vi "Report - Parse Data to TDMS (SubVI).vi"(8 "error in (no error)":errorcluster, 11 "Cluster":T1) -> (0 "error out":errorcluster, 3 "Cancel?":bool)   [LabVIEW 2019]
uses:
  Controls/Report - Data Structure.ctl
  <vilib>/httpClient/ClientHandle.ctl
  Controls/JSON - GetData.ctl
  <vilib>/httpClient/POSTBuffer.vi
  <vilib>/httpClient/LabVIEWHTTPClient.lvlib
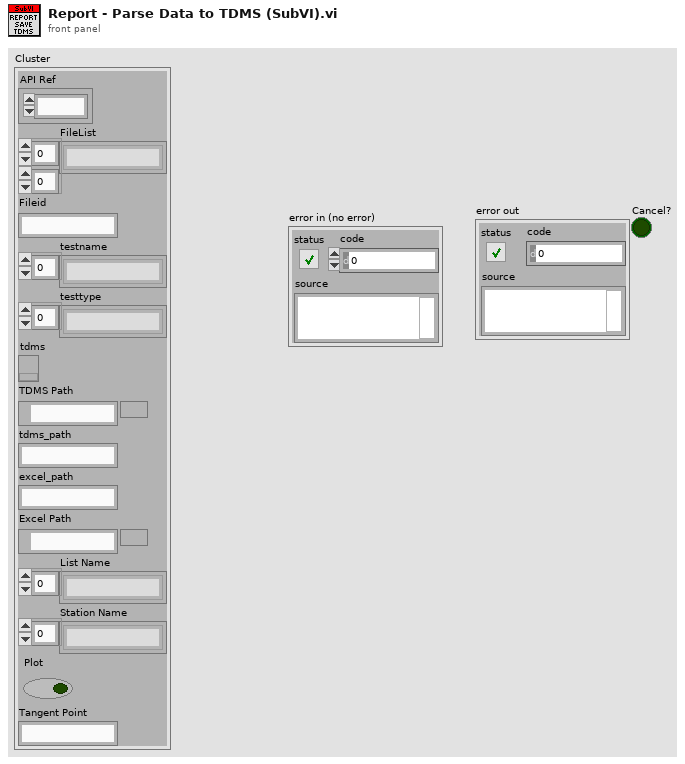
[diagram p1: front panel]
types:
  T1 = typedef "Report - Data Structure.ctl" = cluster{"API Ref":T2, "FileList":string[][], "Fileid":string, "testname":string[], "testtype":string[], "tdms":refnum<k34>, "TDMS Path":path, "tdms_path":string, "excel_path":string, "Excel Path":path, "List Name":string[], "Station Name":string[], "Plot":bool, "Tangent Point":string}
  T2 = typedef "LabVIEWHTTPClient.lvlib/ClientHandle.ctl" = refnum<k1>
  T3 = cluster{"status":string, "data":cluster{"id":string, "created_date":string, "testname":string, "jobno":string, "jobdesc":string, "sampleid":string, "date":string, "specimentno":string, "depth":string, "height":string, "diameter":string, "weight":string, "done":string}[]}
  T4 = cluster{"id":string, "created_date":string, "testname":string, "jobno":string, "jobdesc":string, "sampleid":string, "date":string, "specimentno":string, "depth":string, "height":string, "diameter":string, "weight":string, "done":string}[]
  T5 = cluster{"id":string, "created_date":string, "testname":string, "jobno":string, "jobdesc":string, "sampleid":string, "date":string, "specimentno":string, "depth":string, "height":string, "diameter":string, "weight":string, "done":string}
  T6 = cluster{"testtype":u16, "testname":string, "fileid":string}
  T7 = typedef "JSON - GetData.ctl" = cluster{"status":string, "data":cluster{"timestamp":string, "elapsetime":string, "testname":string, "testtype":u16, "data":string[]}[]}
  T8 = cluster{"timestamp":string, "elapsetime":string, "testname":string, "testtype":u16, "data":string[]}[]
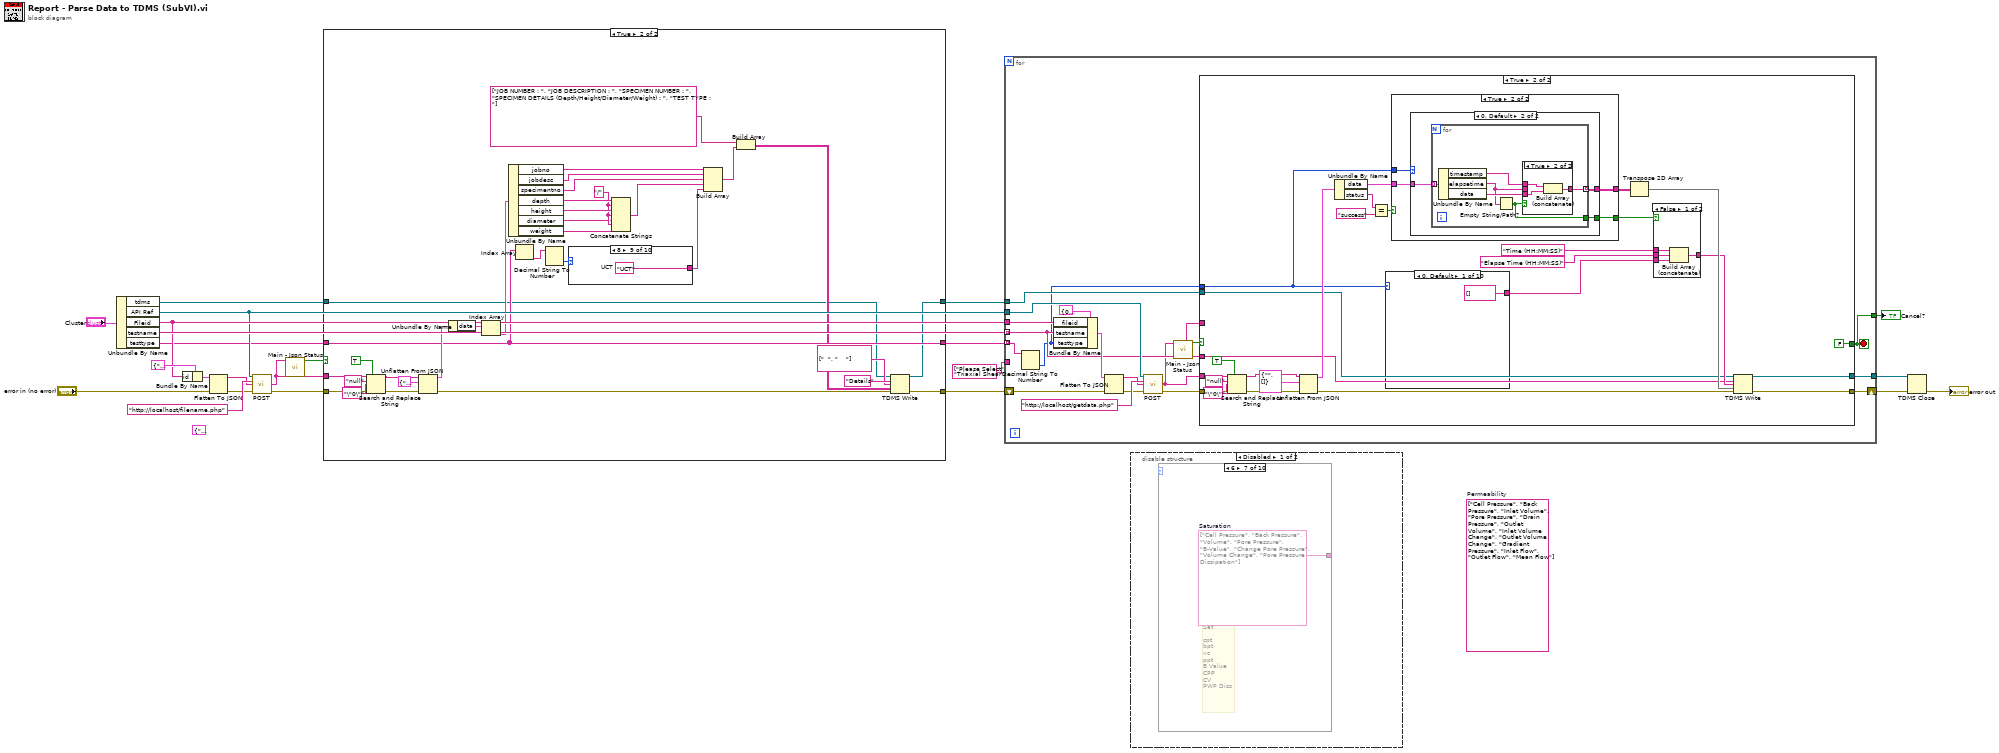
[diagram p0: block diagram]
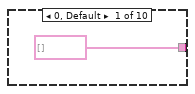
[diagram p2: hidden frame]
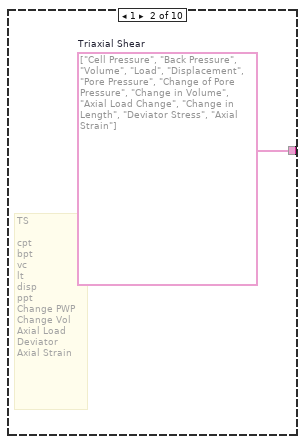
[diagram p3: hidden frame]
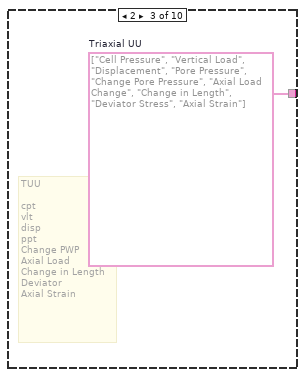
[diagram p4: hidden frame]
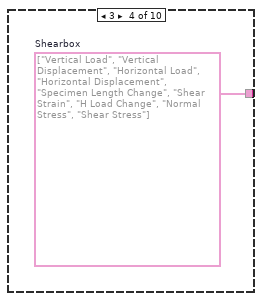
[diagram p5: hidden frame]
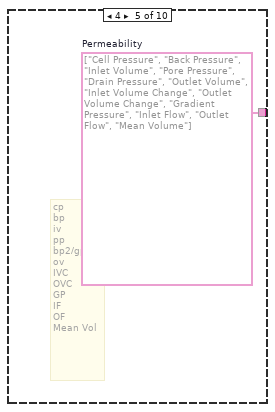
[diagram p6: hidden frame]
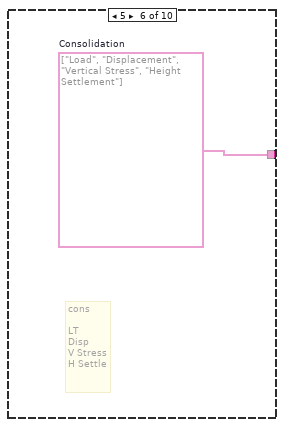
[diagram p7: hidden frame]
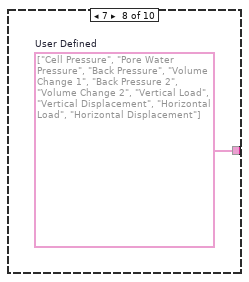
[diagram p8: hidden frame]
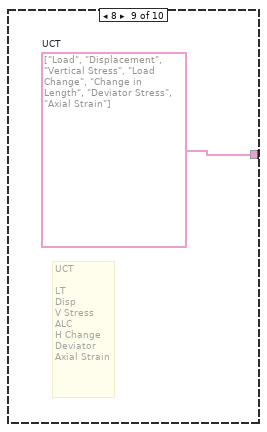
[diagram p9: hidden frame]
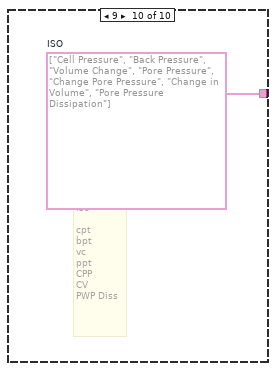
[diagram p10: hidden frame]
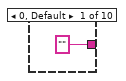
[diagram p13: hidden frame]
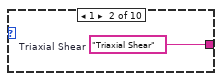
[diagram p14: hidden frame]
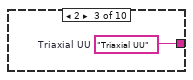
[diagram p15: hidden frame]
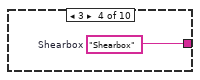
[diagram p16: hidden frame]
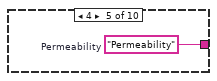
[diagram p17: hidden frame]
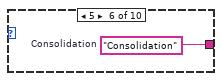
[diagram p18: hidden frame]
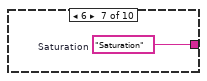
[diagram p19: hidden frame]
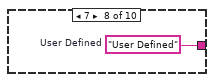
[diagram p20: hidden frame]
diagram:
  (unwired) string[] ["Cell Pressure", "Back Pressure", "Inlet Volume", "Pore Pressure", "Drain Pressure", "Outlet Volume", "Inlet Volume Change", "Outlet Volume Change", "Gradient Pressure", "Inlet Flow", "Outlet Flow", "Mean Flow"]  # Permeability
  (unwired) cluster{"action":string} {"action"="read_all"}
  n1 = Unbundle By Name("Cluster") -> ("tdms"=w4:refnum<k34>, "API Ref"=w5:T2, "Fileid"=w10:string, "testname"=w21:string[], "testtype"=w3:string[])
  n2 = Bundle By Name(cluster=cluster{"action":string, "id":string} {"action"="read_by_id", "id"="2"}, "id"=w10) -> (w14:cluster{"action":string, "id":string})
  n3 = Flatten To JSON(anything=w14, error in (no error)="error in (no error)") -> (JSON string=w15:string, 11:w12:errorcluster)  [unwired: 1 in]
  n4 = call-poly <vilib>:"POST.vi"("client handle"=w5, "url"="http://localhost/filename.php", "buffer"=w15, "error in (no error)"=w12) -> ("body"=w7:string, "error out"=w8:errorcluster)  [unwired: 8 in, 2 out]
  n5 = call "Main - Json Status.vi"("json"=w7) -> ("Success?"=w6:bool)  [unwired: 9 in, 1 out]
  n6 = case shown="True" w6 {
    tunnel: [w26 w32] -> w9
    tunnel: w8 -> [w26 w55]
    tunnel: w7 -> [_ w53]
    tunnel: w4 -> [w24 w27]
    tunnel: w3 -> [w25 w48]
    tunnel: [w24 w31] -> w2
    tunnel: [w25 w48] -> w1
    frame False {
    }
    frame True {
      w45 = "/" ("string")
      n7 = Search and Replace String(replace all?=TRUE ("replace all? (F)"), input string=w53, search string="null", replace string="\"0\"" ("replace string (\"\")"), error in=w55) -> (result string=w52:string, error out=w54:errorcluster)  [unwired: 3 in, 2 out]
      n8 = Unflatten From JSON(JSON string=w52, type and defaults=T3 {"status"="read_all", "data"=[]}, error in (no error)=w54) -> (value=w51:T3, error out=w33:errorcluster)  [unwired: 4 in]
      n9 = Unbundle By Name(w51) -> ("data"=w50:T4)
      n10 = Index Array(array=w50) -> (element=w49:T5)  [unwired: 1 in]
      n11 = Unbundle By Name(w49) -> ("jobno"=w40:string, "jobdesc"=w39:string, "specimentno"=w38:string, "depth"=w47:string, "height"=w46:string, "diameter"=w44:string, "weight"=w43:string)
      n12 = Index Array(array=w48) -> (element=w42:string)  [unwired: 1 in]
      n13 = Decimal String To Number(string=w42) -> (number=w41:i32)  [unwired: 2 in, 1 out]
      n14 = case shown="8" w41 {
        tunnel: ["" w61 w62 w63 w64 w65 w66 w67 w68 w69] -> w36
        frame 0, Default {
        }
        frame 1 {
          w61 = "Triaxial Shear"  # Triaxial Shear
        }
        frame 2 {
          w62 = "Triaxial UU"  # Triaxial UU
        }
        frame 3 {
          w63 = "Shearbox"  # Shearbox
        }
        frame 4 {
          w64 = "Permeability"  # Permeability
        }
        frame 5 {
          w65 = "Consolidation"  # Consolidation
        }
        frame 6 {
          w66 = "Saturation"  # Saturation
        }
        frame 7 {
          w67 = "User Defined"  # User Defined
        }
        frame 8 {
          w68 = "UCT"  # UCT
        }
        frame 9 {
          w69 = "Iso Consolidation"  # Iso
        }
      }
      n15 = Concatenate Strings(w47, w45, w46, w45, w44, w45, w43) -> (w37:string)
      n16 = Build Array(w40, w39, w38, w37, w36) -> (w34:string[])
      n17 = Build Array(string[] ["JOB NUMBER : ", "JOB DESCRIPTION : ", "SPECIMEN NUMBER : ", "SPECIMEN DETAILS (Depth/Height/Diameter/Weight) : ", "TEST TYPE : "], w34) -> (w28:string[][])
      n18 = TDMS Write(0:w27, 5:"Details" ("group name in (Untitled)"), 7:string[] ["  ", "    "] ("channel name(s) in (Untitled)"), 9:w28, 11:w33) -> (4:w31:refnum<k34>, 15:w32:errorcluster)  [unwired: 1 in, 2 out]
    }
  }
  n19 = for {
    tunnel: w21 -> [w79] mode=indexing
    tunnel: w1 -> [w75] mode=indexing
    tunnel: w10 -> [w86]
    tunnel: w5 -> [w81]
    tunnel: string[] ["Please Select", "Triaxial Shear", "Triaxial UU", "Shearbox", "Permeability", "Consolidation", "Saturation", "User Defined"] ("Strings []") -> [_]
    shift-right: [w78] -> w20
    shift-left: w9 -> [w85]
    tunnel: w2 -> [w80]
    tunnel: [w77] -> w18
    tunnel: [w70] -> w17
    stop <- w70 stop-if-true
    n20 = Decimal String To Number(string=w75) -> (number=w74:i32)  [unwired: 2 in, 1 out]
    n21 = Bundle By Name(cluster=T6 {"testtype"=0, "testname"="", "fileid"=""}, "fileid"=w86, "testname"=w79, "testtype"=w74) -> (w87:T6)
    n22 = Flatten To JSON(anything=w87, error in (no error)=w85) -> (JSON string=w82:string, 11:w83:errorcluster)  [unwired: 1 in]
    n23 = call-poly <vilib>:"POST.vi"("client handle"=w81, "url"="http://localhost/getdata.php", "buffer"=w82, "error in (no error)"=w83) -> ("body"=w73:string, "error out"=w76:errorcluster)  [unwired: 8 in, 2 out]
    n24 = call "Main - Json Status.vi"("json"=w73) -> ("Success?"=w72:bool, "message"=w71:string)  [unwired: 9 in]
    n25 = case shown="True" w72 {
      tunnel: w80 -> [w96 w112]
      tunnel: w79 -> [_ w111]
      tunnel: [w97 w110] -> w78
      tunnel: [w96 w99] -> w77
      tunnel: w76 -> [w97 w109]
      tunnel: w74 -> [_ w98]
      tunnel: w73 -> [w92 w103]
      tunnel: w71 -> [w89 _]
      tunnel: [w93 FALSE ("T button?")] -> w70
      frame False {
        n26 = Concatenate Strings(w92, " " ("string"), w89) -> (w90:string)
        n27 = Two Button Dialog(message=w90, 1:"Proceed without this data" ("F button name (\"Cancel\")"), 2:"Cancel report generation" ("T button name (\"OK\")")) -> (T button?=w93:bool)
      }
      frame True {
        n28 = Search and Replace String(replace all?=TRUE ("replace all? (F)"), input string=w103, search string="null", replace string="\"0\"" ("replace string (\"\")"), error in=w109) -> (result string=w107:string, error out=w108:errorcluster)  [unwired: 3 in, 2 out]
        n29 = Unflatten From JSON(JSON string=w107, type and defaults=T7 {"status"="", "data"=[]}, error in (no error)=w108) -> (value=w119:T7, error out=w113:errorcluster)  [unwired: 4 in]
        n30 = Unbundle By Name(w119) -> ("data"=w122:T8, "status"=w121:string)
        n31 = Equal?(x=w121, y="success") -> (x = y?=w123:bool)
        n32 = case shown="0, Default" w98 {
          tunnel: [string[] [] w133 w134 w135 w136 w137 w138 w139 w140 w141] -> w100
          frame 0, Default {
          }
          frame 1 {
            w133 = string[] ["Cell Pressure", "Back Pressure", "Volume Change", "Load", "Displacement", "Pore Pressure", "Change of Pore Pressure", "Change in Volume", "Axial Load Change", "Change in Length", "Deviator Stress", "Axial Strain"]  # Triaxial Shear
          }
          frame 2 {
            w134 = string[] ["Cell Pressure", "Vertical Load", "Displacement", "Pore Pressure", "Change Pore Pressure", "Axial Load Change", "Change in Length", "Deviator Stress", "Axial Strain"]  # Triaxial UU
          }
          frame 3 {
            w135 = string[] ["Vertical Load", "Vertical Displacement", "Horizontal Load", "Horizontal Displacement", "Specimen Length Change", "Shear Strain", "H Load Change", "Normal Stress", "Shear Stress"]  # Shearbox
          }
          frame 4 {
            w136 = string[] ["Cell Pressure", "Back Pressure", "Inlet Volume", "Pore Pressure", "Drain Pressure", "Outlet Volume", "Inlet Volume Change", "Outlet Volume Change", "Gradient Pressure", "Inlet Flow", "Outlet Flow", "Mean Flow"]  # Permeability
          }
          frame 5 {
            w137 = string[] ["Load", "Displacement", "Vertical Stress", "Height Settlement", "Total Height Settlement"]  # Consolidation
          }
          frame 6 {
            w138 = string[] ["Cell Pressure", "Back Pressure", "Sample Volume", "Pore Pressure", "B-Value", "Pore Pressure Change", "Sample Volume Change"]  # Saturation
          }
          frame 7 {
            w139 = string[] ["Cell Pressure", "Pore Water Pressure", "Back Pressure", "Volume Change 1", "Back Pressure 2", "Volume Change 2", "Vertical Load", "Vertical Displacement", "Horizontal Load", "Horizontal Displacement"]  # User Defined
          }
          frame 8 {
            w140 = string[] ["Load", "Displacement", "Vertical Stress", "Load Change", "Change in Length", "Deviator Stress", "Axial Strain"]  # UCT
          }
          frame 9 {
            w141 = string[] ["Cell Pressure", "Back Pressure", "Sample Volume", "Pore Pressure", "Pore Pressure Change", "Sample Volume Change", "Pore Pressure Dissipation"]  # Iso
          }
        }
        n33 = case shown="True" w123 {
          tunnel: w122 -> [_ w147]
          tunnel: [string[][] [] w146] -> w115
          tunnel: [FALSE w145] -> w117
          tunnel: w98 -> [_ w144]
          frame False {
          }
          frame True {
            n34 = case shown="0, Default" w144 {
              tunnel: w147 -> [w151 w172]
              tunnel: [w150 w171] -> w146
              tunnel: [w149 w170] -> w145
              frame 5 {
                n35 = for {
                  tunnel: w151 -> [w160] mode=indexing
                  tunnel: [w158] -> w150 mode=indexing if=w153
                  tunnel: [w157] -> w149
                  shift-right: [w154] -> _
                  shift-left: "" -> [w155]
                  n36 = Unbundle By Name(w160) -> ("timestamp"=w159:string, "elapsetime"=w154:string, "data"=w156:string[])
                  n37 = Empty String/Path?(string/path=w154) -> (empty?=w157:bool)
                  n38 = Not Equal?(x=w155, y=w154) -> (x != y?=w152:bool)
                  n39 = case shown="False" w157 {
                    tunnel: w159 -> [w165 w169]
                    tunnel: w156 -> [w162 w167]
                    tunnel: [w164 w168] -> w158
                    tunnel: w154 -> [w163 _]
                    tunnel: [w161 TRUE] -> w153
                    tunnel: w152 -> [w161 _]
                    frame False {
                      n40 = Build Array (concatenate)(w165, w163, w162) -> (w164:string[])
                    }
                    frame True {
                      n41 = Build Array (concatenate)(w169, w167) -> (w168:string[])
                    }
                  }
                }
              }
              frame 0, Default {
                n42 = for {
                  tunnel: w172 -> [w178] mode=indexing
                  tunnel: [w176] -> w171 mode=indexing
                  tunnel: [w175] -> w170
                  n43 = Unbundle By Name(w178) -> ("timestamp"=w177:string, "elapsetime"=w173:string, "data"=w174:string[])
                  n44 = Empty String/Path?(string/path=w173) -> (empty?=w175:bool)
                  n45 = case shown="True" w175 {
                    tunnel: w177 -> [w182 w185]
                    tunnel: w174 -> [w179 w183]
                    tunnel: [w181 w184] -> w176
                    tunnel: w173 -> [w180 _]
                    frame False {
                      n46 = Build Array (concatenate)(w182, w180, w179) -> (w181:string[])
                    }
                    frame True {
                      n47 = Build Array (concatenate)(w185, w183) -> (w184:string[])
                    }
                  }
                }
              }
            }
          }
        }
        n48 = Transpose 2D Array(2D array=w115) -> (transposed array=w116:string[][])
        n49 = case shown="False" w117 {
          tunnel: "Time (HH:MM:SS)" ("element") -> [w128 w131]
          tunnel: w100 -> [w125 w129]
          tunnel: [w127 w130] -> w114
          tunnel: "Elapse Time (HH:MM:SS)" ("String") -> [w126 _]
          frame False {
            n50 = Build Array (concatenate)(w128, w126, w125) -> (w127:string[])
          }
          frame True {
            n51 = Build Array (concatenate)(w131, w129) -> (w130:string[])
          }
        }
        n52 = TDMS Write(0:w112, 5:w111, 7:w114, 9:w116, 11:w113) -> (4:w99:refnum<k34>, 15:w110:errorcluster)  [unwired: 1 in, 2 out]
      }
    }
  }
  "Cancel?" <- w17
  n53 = disable-structure shown="Disabled" {
    frame Disabled {
      n54 = case shown="6" {
        selector: _ -> [_ _ _ _ _ _ _ _ _ _]
        tunnel: [string[] [] w187 w188 w189 w190 w191 w192 w193 w194 w195] -> _
        frame 0, Default {
        }
        frame 1 {
          w187 = string[] ["Cell Pressure", "Back Pressure", "Volume", "Load", "Displacement", "Pore Pressure", "Change of Pore Pressure", "Change in Volume", "Axial Load Change", "Change in Length", "Deviator Stress", "Axial Strain"]  # Triaxial Shear
          # "TS\n\ncpt\nbpt\nvc\nlt\ndisp\nppt\nChange PWP\nChange Vol\nAxial Load\nDeviator\nAxial Strain"
        }
        frame 2 {
          w188 = string[] ["Cell Pressure", "Vertical Load", "Displacement", "Pore Pressure", "Change Pore Pressure", "Axial Load Change", "Change in Length", "Deviator Stress", "Axial Strain"]  # Triaxial UU
          # "TUU\n\ncpt\nvlt\ndisp\nppt\nChange PWP\nAxial Load\nChange in Length\nDeviator\nAxial Strain"
        }
        frame 3 {
          w189 = string[] ["Vertical Load", "Vertical Displacement", "Horizontal Load", "Horizontal Displacement", "Specimen Length Change", "Shear Strain", "H Load Change", "Normal Stress", "Shear Stress"]  # Shearbox
        }
        frame 4 {
          w190 = string[] ["Cell Pressure", "Back Pressure", "Inlet Volume", "Pore Pressure", "Drain Pressure", "Outlet Volume", "Inlet Volume Change", "Outlet Volume Change", "Gradient Pressure", "Inlet Flow", "Outlet Flow", "Mean Volume"]  # Permeability
          # "cp\nbp\niv\npp\nbp2/gp\nov\nIVC\nOVC\nGP\nIF\nOF\nMean Vol"
        }
        frame 5 {
          w191 = string[] ["Load", "Displacement", "Vertical Stress", "Height Settlement"]  # Consolidation
          # "cons\n\nLT\nDisp\nV Stress\nH Settle"
        }
        frame 6 {
          w192 = string[] ["Cell Pressure", "Back Pressure", "Volume", "Pore Pressure", "B-Value", "Change Pore Pressure", "Volume Change", "Pore Pressure Dissipation"]  # Saturation
          # "Sat\n\ncpt\nbpt\nvc\nppt\nB Value\nCPP\nCV\nPWP Diss"
        }
        frame 7 {
          w193 = string[] ["Cell Pressure", "Pore Water Pressure", "Back Pressure", "Volume Change 1", "Back Pressure 2", "Volume Change 2", "Vertical Load", "Vertical Displacement", "Horizontal Load", "Horizontal Displacement"]  # User Defined
        }
        frame 8 {
          w194 = string[] ["Load", "Displacement", "Vertical Stress", "Load Change", "Change in Length", "Deviator Stress", "Axial Strain"]  # UCT
          # "UCT\n\nLT\nDisp\nV Stress\nALC\nH Change\nDeviator\nAxial Strain"
        }
        frame 9 {
          w195 = string[] ["Cell Pressure", "Back Pressure", "Volume Change", "Pore Pressure", "Change Pore Pressure", "Change in Volume", "Pore Pressure Dissipation"]  # ISO
          # "iso\n\ncpt\nbpt\nvc\nppt\nCPP\nCV\nPWP Diss"
        }
      }
    }
    frame Enabled {
    }
  }
  n55 = TDMS Close(8:w20, 11:w18) -> (0:→"error out":errorcluster)  [unwired: 1 out]
